vi "Inverse_Kinematics_3_arms.vi"(8 "L 2":dbl(slide)=85.0 scale=0.0..200.0, 9 "L 1":dbl(slide)=77.5 scale=0.0..200.0, 11 "end effector":cluster{dbl, dbl}={160.0, 0.0} {"?" format="%.1f"; "?" format="%#.1f"}) -> (0 "Angle 2":dbl(knob)=69.06594950947611 scale=-90.0..90.0, 1 "Angle1":dbl(knob)=-132.16801747912513 scale=-90.0..90.0, 3 "Angle 3":dbl(knob)=63.10206796964901 scale=-90.0..90.0)   [LabVIEW 2024]
panel:
  out "end effector 2":cluster{dbl, dbl}={160.0, 5.684341886080802e-14} {"?" format="%.1f"; "?" format="%#.1f"}
  # "mm"
  # "mm"
  # "mm"
  # "mm"
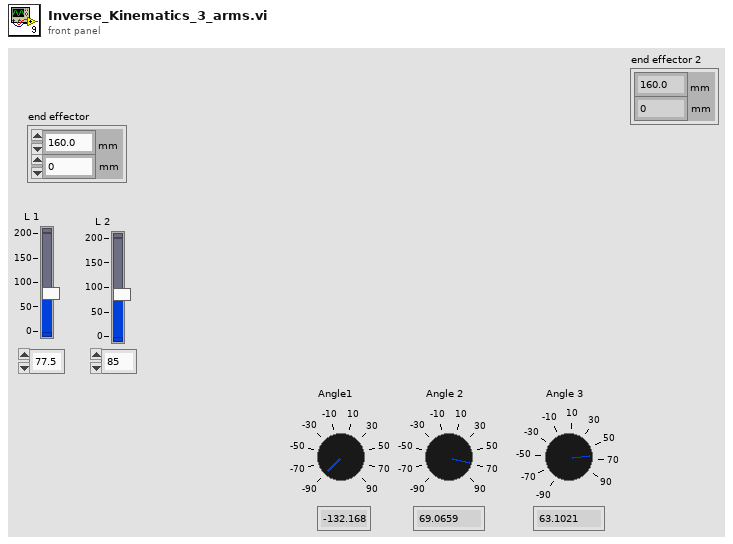
[diagram p1: front panel]
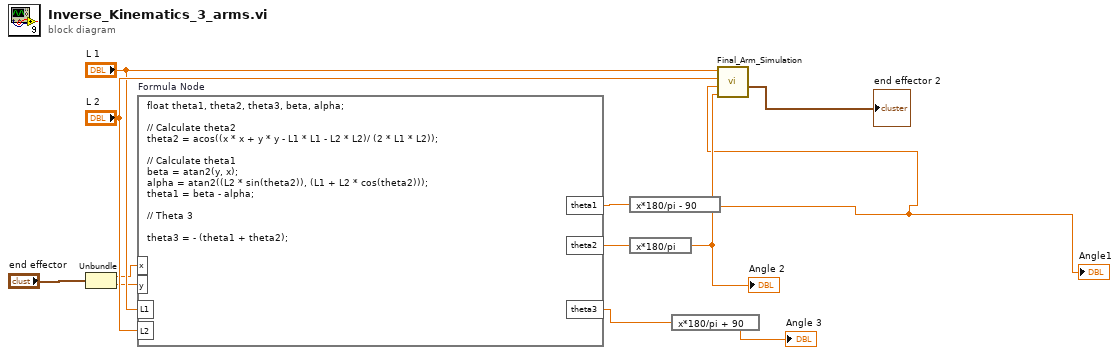
[diagram p0: block diagram]
diagram:
  n1 = Unbundle("end effector") -> (w4:dbl, w5:dbl)
  n2 = formula code="float theta1, theta2, theta3, beta, alpha;\n\n// Calculate theta2\ntheta2 = acos((x * x + y * y - L1 * L1 - L2 * L2)/ (2 * L1 * L2));\n\n// Calculate theta1\nbeta = atan2(y, x);\nalpha = atan2((L2 * sin(theta2)), (L1 + L2 * cos(theta2)));\ntheta1 = beta - alpha;\n\n// Theta 3\n\ntheta3 = - (theta1 + theta2);"("L1"="L 1", "L2"="L 2", "x"=w4, "y"=w5) -> ("theta1"=w10:dbl, "theta2"=w8:dbl, "theta3"=w3:dbl)
  n3 = expression code="x*180/pi - 90"(w10) -> (w1:dbl)
  "Angle1" <- w1
  n4 = expression code="x*180/pi"(w8) -> (w9:dbl)
  "Angle 2" <- w9
  n5 = expression code="x*180/pi + 90"(w3) -> (→"Angle 3":dbl)
  n6 = call "Final_Arm_Simulation.vi"("Angle 2"=w9, "Angle1"=w1, "L 2"="L 2", "L 1"="L 1") -> ("end effector"=→"end effector 2":cluster{dbl, dbl})  [unwired: 6 in, 1 out]
